vi "Set Data Type Buffers.vi"(10 "data type buffers":T1, 11 "Transceiver Thread in":refnum<class "Plugin Thread.lvclass">) -> (3 "Transceiver Thread out":refnum<class "Plugin Thread.lvclass">)   [LabVIEW 2017, in "DSF Core.lvlib" / "Plugin Thread.lvclass"]
uses:
  Plugin Thread.lvclass
  Typedefs/DSF Runtime Type Buffers.ctl
  Plugin Thread.lvclass/Plugin Thread.ctl
  DSF Core.lvlib
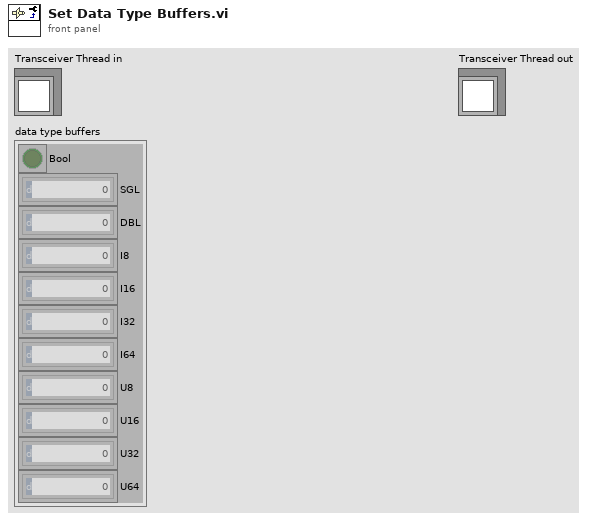
[diagram p1: front panel]
types:
  T1 = typedef "DSF Core.lvlib/DSF Runtime Type Buffers.ctl" = cluster{"Bool":bool[], "SGL":sgl[], "DBL":dbl[], "I8":i8[], "I16":i16[], "I32":i32[], "I64":i64[], "U8":u8[], "U16":u16[], "U32":u32[], "U64":u64[]}
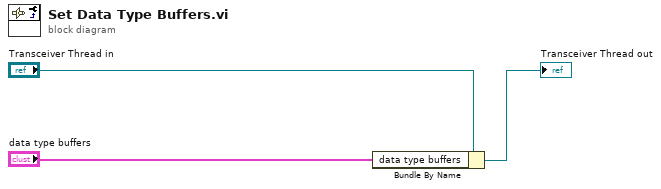
[diagram p0: block diagram]
diagram:
  n1 = Bundle By Name(cluster="Transceiver Thread in", "data type buffers"="data type buffers") -> (→"Transceiver Thread out":refnum<class "Plugin Thread.lvclass">)
